vi "casg.vi"(0 "IP adress":string="192.109.209.229", 1 "stop":bool, 2 "Channel":u8(ring)=1 items=["1", "2", "3", "4", "5", "6", "7", "8", "9", "10", "11", "12", "13", "14", "15", "16"], 4 "Exit":bool, 5 "Start":bool, 6 "Draw":enum16{"Ewe(t)", "I(t)"}(ring)) -> (7 "XY Graph":cluster{"Data 101":sgl[], "Data 101":sgl[]}(graph)={"Data 101"=[0.0, 0.01, 0.02, 0.03, 0.04, 0.049999997, 0.06, 0.07, 0.08, 0.089999996, 0.099999994, 0.11, 0.12, 0.13, 0.14, 0.14999999, 0.16, 0.17, 0.17999999, 0.19, 0.19999999, 0.21, 0.22, 0.22999999, 0.24, 0.25, 0.26, 0.26999998, 0.28, 0.29, 0.29999998, 0.31, 0.32, 0.32999998, 0.34, 0.35, 0.35999998, 0.37, 0.38, 0.39, 0.39999998, 0.41, 0.42, 0.42999998, 0.44, 0.45, 0.45999998, 0.47, 0.48, 0.48999998, 0.5, 0.51, 0.52, 0.53, 0.53999996, 0.55, 0.56, 0.57, 0.58, 0.59, 0.59999996, 0.61, 0.62, 0.63, 0.64, 0.65, 0.65999997, 0.66999996, 0.68, 0.69, 0.7, 0.71, 0.71999997, 0.72999996, 0.74, 0.75, 0.76, 0.77, 0.78, 0.78999996, 0.79999995, 0.81, 0.82, 0.83, 0.84, 0.84999996, 0.85999995, 0.87, 0.88, 0.89, 0.9, 0.90999997, 0.91999996, 0.92999995, 0.94, 0.95, 0.96, 0.96999997, 0.97999996, 0.98999995, 1.0, 1.01, 1.02, 1.03, 1.04, 1.05, 1.06, 1.0699999, 1.0799999, 1.0899999, 1.1, 1.11, 1.12, 1.13, 1.14, 1.15, 1.16, 1.17, 1.18, 1.1899999, 1.1999999, 1.2099999, 1.22, 1.23, 1.24, 1.25, 1.26, 1.27, 1.28, 1.29, 1.3, 1.31, 1.3199999, 1.3299999, 1.3399999, 1.35, 1.36, 1.37, 1.38, 1.39, 1.4, 1.41, 1.42, 1.43, 1.4399999, 1.4499999, 1.4599999, 1.4699999, 1.48, 1.49, 1.5, 1.51, 1.52, 1.53, 1.54, 1.55, 1.56, 1.5699999, 1.5799999, 1.5899999, 1.5999999, 1.61, 1.62, 1.63, 1.64, 1.65, 1.66, 1.67, 1.68, 1.6899999, 1.6999999, 1.7099999, 1.7199999, 1.7299999, 1.74, 1.75, 1.76, 1.77, 1.78, 1.79, 1.8, 1.81, 1.8199999, 1.8299999, 1.8399999, 1.8499999, 1.8599999, 1.87, 1.88, 1.89, 1.9, 1.91, 1.92, 1.93, 1.9399999, 1.9499999, 1.9599999, 1.9699999, 1.9799999, 1.9899999, 2.0, 2.01, 2.02, 2.03, 2.04, 2.05, 2.06, 2.07, 2.08, 2.09, 2.1, 2.11, 2.12, 2.1299999, 2.1399999, 2.1499999, 2.1599998, 2.1699998, 2.1799998, 2.19, 2.2, 2.21, 2.22, 2.23, 2.24, 2.25, 2.26, 2.27, 2.28, 2.29, 2.3, 2.31, 2.32, 2.33, 2.34, 2.35, 2.36, 2.37, 2.3799999, 2.3899999, 2.3999999, 2.4099998, 2.4199998, 2.4299998, 2.44, 2.45, 2.46, 2.47, 2.48, 2.49, 2.5, 2.51, 2.52, 2.53, 2.54, 2.55, 2.56, 2.57, 2.58, 2.59, 2.6, 2.61, 2.62, 2.6299999, 2.6399999, 2.6499999, 2.6599998, 2.6699998, 2.6799998, 2.6899998, 2.7, 2.71, 2.72, 2.73, 2.74, 2.75, 2.76, 2.77, 2.78, 2.79, 2.8, 2.81, 2.82, 2.83, 2.84, 2.85, 2.86, 2.87, 2.8799999, 2.8899999, 2.8999999, 2.9099998, 2.9199998, 2.9299998, 2.9399998, 2.9499998, 2.96, 2.97, 2.98, 2.99, 3.0], "Data 101"=array[301 elements]}, 8 "Number of points":i32=301)   [LabVIEW 2014]
uses:
  LLB/dll_Functions.llb/CASGParameters.ctl
panel:
  in  "Display Parameters?":bool caption="Display Parameters"
  out "DllPath":path caption="DLL Path"
  out "LibVersion":string caption="DLL Version"
  in  "CASG Parameters":T1={"Ii"=0.0, "Ii_vs_initial"=TRUE, "Steps"=[{"I1_vs_initial"=FALSE, "I1"=0.0005, "Period_number"=3, "Fs"=1.0, "Record_every_dE"=1.0, "Record_every_dT"=0.01, "I2_vs_initial"=TRUE, "I2"=0.0}, {"I1_vs_initial"=FALSE, "I1"=0.002, "Period_number"=4, "Fs"=10.0, "Record_every_dE"=0.1, "Record_every_dT"=0.001, "I2_vs_initial"=TRUE, "I2"=0.0}], "Step_number"=1, "N_Cycles"=0, "I_Range"=8, "Bandwidth"=5, "em"=1, "ce"=0, "tb"=5e-05} {"tb" min=5e-05 max=1 format="%^_3e"; "Step_number" min=0 max=99; "Steps"."I2" min=-150 max=150 format="%^_3e"; "Steps"."Record_every_dT" min=0 format="%.2e"; "Steps"."Record_every_dE" min=0 format="%.2e"; "Steps"."Fs" min=1e-05 max=1000000 format="%.2e"; "Steps"."Period_number" min=1; "Steps"."I1" min=-150 max=150 format="%^_3e"; "ce" items=["Standard", "CE to ground"]; "Ii" min=-10 max=10 format="%.5f"; "I_Range" items=["1pA", "1nA", "10nA", "100nA", "1µA", "10µA", "100µA", "1mA", "10mA", "100mA", "1A", "Booster"]; "Bandwidth" items=["1"=1, "2"=2, "3"=3, "4"=4, "5"=5, "6"=6, "7"=7, "8"=8, "9"=9]; "N_Cycles" min=0 max=1000 step=1}
  out "Exit 2":bool=TRUE
  out "Data 169":sgl[][](array[numeric])=[[0.0, 0.0009888702, 0.0, 1.0], [0.01, 0.036624238, 3.9297032e-05, 1.0], [0.02, 0.06807284, 6.7561894e-05, 1.0], [0.03, 0.09920054, 0.000100410245, 1.0], [0.04, 0.13097005, 0.00013096684, 1.0], [0.049999997, 0.15985142, 0.00016075955, 1.0], [0.06, 0.1896955, 0.00018902442, 1.0], [0.07, 0.21889777, 0.00021958101, 1.0], [0.08, 0.24681643, 0.00024708195, 1.0], [0.089999996, 0.27345148, 0.00027611072, 1.0], [0.099999994, 0.29976562, 0.00029826426, 1.0], [0.11, 0.32351252, 0.0003250013, 1.0], [0.12, 0.3475803, 0.00034791877, 1.0], [0.13, 0.37100634, 0.00037083623, 1.0], [0.14, 0.3905815, 0.00039069803, 1.0], [0.14999999, 0.41015664, 0.00041132374, 1.0], [0.16, 0.42748544, 0.00042889378, 1.0], [0.17, 0.44353065, 0.00044493595, 1.0], [0.17999999, 0.45893404, 0.0004609782, 1.0], [0.19, 0.4704866, 0.00047396476, 1.0], [0.19999999, 0.48236004, 0.00048313173, 1.0], [0.21, 0.49070355, 0.0004892431, 1.0], [0.22, 0.49712163, 0.0004999379, 1.0], [0.22999999, 0.50193524, 0.00050222967, 1.0], [0.24, 0.50514424, 0.0005068131, 1.0], [0.25, 0.50546515, 0.0005060492, 1.0], [0.26, 0.5045025, 0.00050452136, 1.0], [0.26999998, 0.5012934, 0.0005029935, 1.0], [0.28, 0.49615893, 0.00049917394, 1.0], [0.29, 0.48974085, 0.0004892431, 1.0], [0.29999998, 0.48171824, 0.0004846596, 1.0], [0.31, 0.4708075, 0.00047396476, 1.0], [0.32, 0.45861316, 0.00045868644, 1.0], [0.32999998, 0.44417247, 0.0004456999, 1.0], [0.34, 0.42844817, 0.00043042158, 1.0], [0.35, 0.41047752, 0.00041132374, 1.0], [0.35999998, 0.39026058, 0.00039146192, 1.0], [0.37, 0.37100634, 0.00037083623, 1.0], [0.38, 0.34725943, 0.0003486827, 1.0], [0.39, 0.32479614, 0.00032576523, 1.0], [0.39999998, 0.2988029, 0.00030131993, 1.0], [0.41, 0.27441418, 0.00027687466, 1.0], [0.42, 0.24777915, 0.00024860978, 1.0], [0.42999998, 0.21953958, 0.00021881709, 1.0], [0.44, 0.1900164, 0.00018978832, 1.0], [0.45, 0.16017233, 0.00015999563, 1.0], [0.45999998, 0.13129096, 0.00013173078, 1.0], [0.47, 0.10016325, 0.00010346591, 1.0], [0.48, 0.06871465, 6.8325804e-05, 1.0], [0.48999998, 0.036624238, 3.8533115e-05, 1.0], [0.5, 0.0058174427, 7.212594e-06, 1.0], [0.51, -0.025310256, -2.334401e-05, 1.0], [0.52, -0.056758855, -5.542844e-05, 1.0], [0.53, -0.08788655, -8.674896e-05, 1.0], [0.53999996, -0.11805154, -0.000117305564, 1.0], [0.55, -0.14853743, -0.00014862607, 1.0], [0.56, -0.1780606, -0.00017765485, 1.0], [0.57, -0.20758379, -0.00020668362, 1.0], [0.58, -0.23582333, -0.00023265673, 1.0], [0.59, -0.26245838, -0.00026092157, 1.0], [0.59999996, -0.28748888, -0.0002861308, 1.0], [0.61, -0.31348214, -0.0003128678, 1.0], [0.62, -0.3362663, -0.0003365492, 1.0], [0.63, -0.3596923, -0.0003571749, 1.0], [0.64, -0.37990928, -0.00037627274, 1.0], [0.65, -0.39852172, -0.00039689848, 1.0], [0.65999997, -0.41552964, -0.00041523244, 1.0], [0.66999996, -0.43189573, -0.00043051073, 1.0], [0.68, -0.44665733, -0.0004450251, 1.0], [0.69, -0.45917258, -0.00045724778, 1.0], [0.7, -0.46912062, -0.00046794256, 1.0], [0.71, -0.4774641, -0.00047787346, 1.0], [0.71999997, -0.4851658, -0.0004839848, 1.0], [0.72999996, -0.4899794, -0.0004893322, 1.0], [0.74, -0.49415115, -0.00049162394, 1.0], [0.75, -0.49447203, -0.0004931517, 1.0], [0.76, -0.49447203, -0.00049086, 1.0], [0.77, -0.49062118, -0.0004893322, 1.0], [0.78, -0.48484492, -0.00048322088, 1.0], [0.78999996, -0.47874773, -0.00047940132, 1.0], [0.79999995, -0.47040424, -0.00046870648, 1.0], [0.81, -0.4588517, -0.00045801167, 1.0], [0.82, -0.44665733, -0.00044578905, 1.0], [0.83, -0.43317935, -0.00043203856, 1.0], [0.84, -0.41681325, -0.00041446852, 1.0], [0.84999996, -0.3991635, -0.0003984263, 1.0], [0.85999995, -0.3802302, -0.0003785645, 1.0], [0.87, -0.35937142, -0.0003587027, 1.0], [0.88, -0.33754992, -0.0003334935, 1.0], [0.89, -0.31444484, -0.0003121039, 1.0], [0.9, -0.2884516, -0.0002876586, 1.0], [0.90999997, -0.26310018, -0.0002616855, 1.0], [0.91999996, -0.23550244, -0.00023494849, 1.0], [0.92999995, -0.20758379, -0.0002059197, 1.0], [0.94, -0.17870241, -0.00017841876, 1.0], [0.95, -0.15014194, -0.00014938999, 1.0], [0.96, -0.11901425, -0.000117305564, 1.0], [0.96999997, -0.08884926, -8.598504e-05, 1.0], [0.97999996, -0.05643795, -5.6192355e-05, 1.0], [0.98999995, -0.025952064, -2.487184e-05, 1.0], [1.0, 0.0058174427, 6.448679e-06, 1.0], [1.01, 0.036303334, 3.8533115e-05, 1.0], [1.02, 0.06711013, 6.908972e-05, 1.0], [1.03, 0.09952144, 0.000100410245, 1.0], [1.04, 0.12936553, 0.00012943902, 1.0], [1.05, 0.16049322, 0.00016075955, 1.0], [1.06, 0.1893746, 0.00019055224, 1.0], [1.0699999, 0.21857686, 0.00022034491, 1.0], [1.0799999, 0.24521191, 0.0002478459, 1.0], [1.0899999, 0.27345148, 0.0002745829, 1.0], [1.1, 0.30008653, 0.000300556, 1.0], [1.11, 0.32447523, 0.0003250013, 1.0], [1.12, 0.3475803, 0.0003502105, 1.0], [1.13, 0.3700436, 0.00037160012, 1.0], [1.14, 0.39026058, 0.00039146192, 1.0], [1.15, 0.41047752, 0.00041285154, 1.0], [1.16, 0.42716455, 0.00042965767, 1.0], [1.17, 0.44353065, 0.00044646382, 1.0], [1.18, 0.45829225, 0.00045868644, 1.0], [1.1899999, 0.4704866, 0.00047090912, 1.0], [1.1999999, 0.48043463, 0.00048083998, 1.0], [1.2099999, 0.49038264, 0.0004892431, 1.0], [1.22, 0.49712163, 0.00049917394, 1.0], [1.23, 0.50161433, 0.0005014657, 1.0], [1.24, 0.5048233, 0.0005060492, 1.0], [1.25, 0.506107, 0.0005060492, 1.0], [1.26, 0.5045025, 0.0005060492, 1.0], [1.27, 0.5012934, 0.00050222967, 1.0], [1.28, 0.49744254, 0.0004953544, 1.0], [1.29, 0.48974085, 0.0004892431, 1.0], [1.3, 0.48203915, 0.00048313173, 1.0], [1.31, 0.4711284, 0.00047243692, 1.0], [1.3199999, 0.45765042, 0.00045792255, 1.0], [1.3299999, 0.44353065, 0.0004456999, 1.0], [1.3399999, 0.42812726, 0.00042889378, 1.0], [1.35, 0.41079843, 0.00041055982, 1.0], [1.36, 0.39090237, 0.00039222583, 1.0], [1.37, 0.37068543, 0.00037236404, 1.0], [1.38, 0.34725943, 0.0003502105, 1.0], [1.39, 0.32543793, 0.00032652915, 1.0], [1.4, 0.2991238, 0.00030131993, 1.0], [1.41, 0.2737724, 0.0002745829, 1.0], [1.42, 0.24649553, 0.0002478459, 1.0], [1.43, 0.21953958, 0.00022034491, 1.0], [1.4399999, 0.1890537, 0.00019131615, 1.0], [1.4499999, 0.16113503, 0.0001638152, 1.0], [1.4599999, 0.13097005, 0.00013020294, 1.0], [1.4699999, 0.10016325, 0.000100410245, 1.0], [1.48, 0.06871465, 6.985364e-05, 1.0], [1.49, 0.03758695, 3.77692e-05, 1.0], [1.5, 0.0058174427, 7.212594e-06, 1.0], [1.51, -0.02563116, -2.4107923e-05, 1.0], [1.52, -0.056758855, -5.542844e-05, 1.0], [1.53, -0.08820745, -8.598504e-05, 1.0], [1.54, -0.11805154, -0.00011806948, 1.0], [1.55, -0.14917924, -0.00014557042, 1.0], [1.56, -0.1780606, -0.00017765485, 1.0], [1.5699999, -0.20662107, -0.0002059197, 1.0], [1.5799999, -0.23486063, -0.00023418457, 1.0], [1.5899999, -0.26277927, -0.00025862985, 1.0], [1.5999999, -0.28748888, -0.0002861308, 1.0], [1.61, -0.3128403, -0.00031133997, 1.0], [1.62, -0.33658722, -0.00033502135, 1.0], [1.63, -0.3577669, -0.00035641095, 1.0], [1.64, -0.37926745, -0.0003785645, 1.0], [1.65, -0.3978799, -0.00039766237, 1.0], [1.66, -0.41681325, -0.00041599633, 1.0], [1.67, -0.43253756, -0.00043203856, 1.0], [1.68, -0.44697824, -0.0004450251, 1.0], [1.6899999, -0.45917258, -0.00045877558, 1.0], [1.6999999, -0.4697624, -0.0004694704, 1.0], [1.7099999, -0.47906864, -0.00047787346, 1.0], [1.7199999, -0.48484492, -0.0004839848, 1.0], [1.7299999, -0.4899794, -0.0004885683, 1.0], [1.74, -0.49383023, -0.00049162394, 1.0], [1.75, -0.49350932, -0.00049391564, 1.0], [1.76, -0.49447203, -0.00049238786, 1.0], [1.77, -0.4899794, -0.00048780435, 1.0], [1.78, -0.48484492, -0.00048474869, 1.0], [1.79, -0.47842684, -0.00047940132, 1.0], [1.8, -0.47040424, -0.00046794256, 1.0], [1.81, -0.4588517, -0.00045953953, 1.0], [1.8199999, -0.44826186, -0.0004450251, 1.0], [1.8299999, -0.43285844, -0.00043127465, 1.0], [1.8399999, -0.41649234, -0.00041676027, 1.0], [1.8499999, -0.39948443, -0.00039460673, 1.0], [1.8599999, -0.37958837, -0.00037780058, 1.0], [1.87, -0.3596923, -0.00035641095, 1.0], [1.88, -0.3362663, -0.000338077, 1.0], [1.89, -0.3128403, -0.00031133997, 1.0], [1.9, -0.2884516, -0.00028918646, 1.0], [1.91, -0.26277927, -0.00026015766, 1.0], [1.92, -0.23646514, -0.00023418457, 1.0], [1.93, -0.20790468, -0.0002059197, 1.0], [1.9399999, -0.1783815, -0.00017841876, 1.0], [1.9499999, -0.14917924, -0.00014938999, 1.0], [1.9599999, -0.11837244, -0.000117305564, 1.0], [1.9699999, -0.08820745, -8.7512875e-05, 1.0], [1.9799999, -0.057721566, -5.4664528e-05, 1.0], [1.9899999, -0.025952064, -2.5635754e-05, 1.0], [2.0, 0.0048547303, 7.212594e-06, 1.0], [2.01, 0.037266046, 3.7005288e-05, 1.0], [2.02, 0.06871465, 6.8325804e-05, 1.0], [2.03, 0.098879635, 9.811849e-05, 1.0], [2.04, 0.12968643, 0.00013249468, 1.0], [2.05, 0.16017233, 0.00016075955, 1.0], [2.06, 0.1896955, 0.00019055224, 1.0], [2.07, 0.21825597, 0.00021958101, 1.0], [2.08, 0.24681643, 0.00024631806, 1.0], [2.09, 0.27280968, 0.000273819, 1.0], [2.1, 0.2991238, 0.0002990282, 1.0], [2.11, 0.32447523, 0.0003242374, 1.0], [2.12, 0.34725943, 0.0003502105, 1.0], [2.1299999, 0.3694018, 0.00036854448, 1.0], [2.1399999, 0.38961875, 0.00039146192, 1.0], [2.1499999, 0.41079843, 0.00040979587, 1.0], [2.1599998, 0.42780635, 0.00043042158, 1.0], [2.1699998, 0.44417247, 0.0004456999, 1.0], [2.1799998, 0.45797133, 0.00045945038, 1.0], [2.19, 0.4698448, 0.00047243692, 1.0], [2.2, 0.48139733, 0.00048389565, 1.0], [2.21, 0.48974085, 0.000490007, 1.0], [2.22, 0.49647984, 0.00049688225, 1.0], [2.23, 0.5022561, 0.00050375744, 1.0], [2.24, 0.5045025, 0.0005060492, 1.0], [2.25, 0.50514424, 0.00050757703, 1.0], [2.26, 0.5048233, 0.0005060492, 1.0], [2.27, 0.5012934, 0.00050375744, 1.0], [2.28, 0.49712163, 0.00049764616, 1.0], [2.29, 0.49038264, 0.0004915348, 1.0], [2.3, 0.48011371, 0.00048389565, 1.0], [2.31, 0.4708075, 0.00047243692, 1.0], [2.32, 0.45797133, 0.00045945038, 1.0], [2.33, 0.44385156, 0.00044493595, 1.0], [2.34, 0.42716455, 0.00042812986, 1.0], [2.35, 0.41047752, 0.00041055982, 1.0], [2.36, 0.39122328, 0.00039298975, 1.0], [2.37, 0.37100634, 0.00037236404, 1.0], [2.3799999, 0.34790123, 0.00034791877, 1.0], [2.3899999, 0.32415432, 0.00032652915, 1.0], [2.3999999, 0.30008653, 0.000300556, 1.0], [2.4099998, 0.2740933, 0.000273819, 1.0], [2.4199998, 0.24681643, 0.0002478459, 1.0], [2.4299998, 0.21825597, 0.00021958101, 1.0], [2.44, 0.1900164, 0.00019055224, 1.0], [2.45, 0.15985142, 0.00016305129, 1.0], [2.46, 0.13032824, 0.00013020294, 1.0], [2.47, 0.09984235, 0.00010117416, 1.0], [2.48, 0.06871465, 6.679798e-05, 1.0], [2.49, 0.038228758, 3.8533115e-05, 1.0], [2.5, 0.0051756343, 6.448679e-06, 1.0], [2.51, -0.02498935, -2.334401e-05, 1.0], [2.52, -0.05643795, -5.6192355e-05, 1.0], [2.53, -0.08852836, -8.8276785e-05, 1.0], [2.54, -0.118693344, -0.00011654164, 1.0], [2.55, -0.14821652, -0.00014633434, 1.0], [2.56, -0.1780606, -0.00017459918, 1.0], [2.57, -0.20694198, -0.00020668362, 1.0], [2.58, -0.23550244, -0.00023418457, 1.0], [2.59, -0.26149565, -0.00026092157, 1.0], [2.6, -0.2878098, -0.00028995035, 1.0], [2.61, -0.3125194, -0.0003121039, 1.0], [2.62, -0.3359454, -0.00033578524, 1.0], [2.6299999, -0.3590505, -0.00035641095, 1.0], [2.6399999, -0.37894657, -0.00037627274, 1.0], [2.6499999, -0.3988426, -0.00039689848, 1.0], [2.6599998, -0.41552964, -0.00041523244, 1.0], [2.6699998, -0.43189573, -0.00043051073, 1.0], [2.6799998, -0.44762003, -0.00044731685, 1.0], [2.6899998, -0.4598144, -0.00045877558, 1.0], [2.7, -0.46912062, -0.00046794256, 1.0], [2.71, -0.47842684, -0.00047710957, 1.0], [2.72, -0.4851658, -0.00048322088, 1.0], [2.73, -0.491263, -0.0004885683, 1.0], [2.74, -0.49350932, -0.0004931517, 1.0], [2.75, -0.49511385, -0.00049391564, 1.0], [2.76, -0.49286753, -0.00049238786, 1.0], [2.77, -0.4919048, -0.0004900961, 1.0], [2.78, -0.4851658, -0.0004839848, 1.0], [2.79, -0.47842684, -0.00047863738, 1.0], [2.8, -0.47040424, -0.0004694704, 1.0], [2.81, -0.45853078, -0.00045953953, 1.0], [2.82, -0.44729912, -0.00044578905, 1.0], [2.83, -0.43253756, -0.00043356637, 1.0], [2.84, -0.41777596, -0.00041446852, 1.0], [2.85, -0.3988426, -0.00039689848, 1.0], [2.86, -0.3802302, -0.0003785645, 1.0], [2.87, -0.3596923, -0.00035793878, 1.0], [2.8799999, -0.33787084, -0.0003334935, 1.0], [2.8899999, -0.31444484, -0.0003121039, 1.0], [2.8999999, -0.2884516, -0.00028842254, 1.0], [2.9099998, -0.26181656, -0.00026092157, 1.0], [2.9199998, -0.23518153, -0.00023418457, 1.0], [2.9299998, -0.20726287, -0.0002059197, 1.0], [2.9399998, -0.17934422, -0.00017841876, 1.0], [2.9499998, -0.14950013, -0.00014862607, 1.0], [2.96, -0.119656056, -0.00011501381, 1.0], [2.97, -0.08884926, -8.522113e-05, 1.0], [2.98, -0.05707976, -5.3136693e-05, 1.0], [2.99, -0.025952064, -2.487184e-05, 1.0], [3.0, 0.004533826, 5.684764e-06, 1.0]] format="%.2f"
  # "Instructions:\nBefore running the VI you must type a valid IP adress that corresponds to the instrument.Then press the Run button to execute this VI.\nWhile this VI is running, choose the available channel, enter the CASG parameters or keep the default values, then press the start button to begin the experience.\nChoose the waveform to draw (Ewe(t) or I(t)). You can stop the measure if you press the stop button and exit the execution if you press the exit button."
  # "Set Ii (A)  vs. previous"
  # "repeat nc times"
  # "with I Range"
  # "bandwidth"
  # "Fs (Hz)"
  # "record every dE (V)"
  # "or every dt (s)"
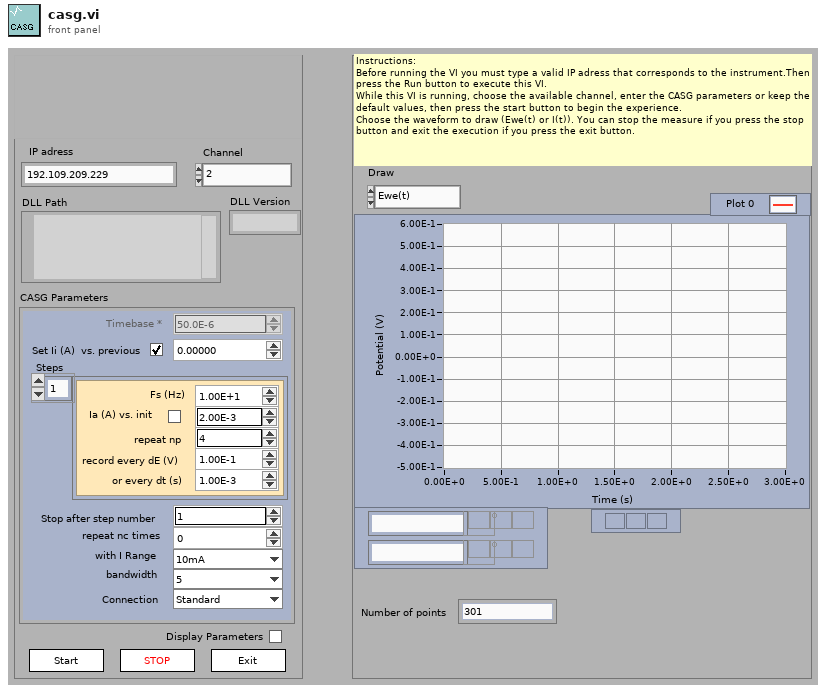
[diagram p1: front panel]
types:
  T1 = typedef "CASGParameters.ctl" = cluster{"Ii":sgl, "Ii_vs_initial":bool, "Steps":cluster{"I1_vs_initial":bool, "I1":sgl, "Period_number":u32, "Fs":sgl, "Record_every_dE":sgl, "Record_every_dT":sgl, "I2_vs_initial":bool, "I2":sgl}[], "Step_number":i32, "N_Cycles":i32, "I_Range":u16, "Bandwidth":u16, "em":u16, "ce":u16, "tb":sgl}
  T2 = cluster{"LibVersion":string, "StringLength":u32, "DllPath":path}
  T3 = cluster{"Channel":i32, "BoardVersion":i32, "BoardSerialCode":i32, "FirmwareCode":i32, "FirmwareVersion":i32, "XilinxVersion":i32, "AmpCode":i32, "NbAmp":i32, "LcBoard":i32, "Zboard":i32, "MuxBoard":i32, "GPRAboard":i32, "MemSize":i32, "MemFilled":i32, "state":i32, "MaxIRange":i32, "MinIRange":i32, "MaxBandwidth":i32, "NbOfTechniques":i32}
  T4 = typedef "TechniqueParameters.ctl" = cluster{"String Label":string, "Type":i32, "Valeur":i32, "Index":i32}
  T5 = cluster{"string before end tag":string, i32, i32, i32}[]
  T6 = cluster{"IRQskipped":i32, "NbRaws":i32, "NbCols":i32, "Technique Index":i32, "TechniqueID":i32, "PrcessIndex":i32, "loop":i32, "StartTime":dbl, "MuxPad":i32}
  T7 = cluster{"State":i32, "MemFilled":i32, "TimeBase":sgl, " Ewe":sgl, " EweRangeMin":sgl, " EweRangeMax":sgl, "Ece":sgl, "EceRangeMin":sgl, "EceRangeMax":sgl, "Eoverflow":i32, "I":sgl, "IRange":i32, "Ioverflow":i32, "ElapsedTime":sgl, "Freq":sgl, "Rcomp":sgl, "Saturation":sgl, "OptErr":i32, "OptPos":i32}
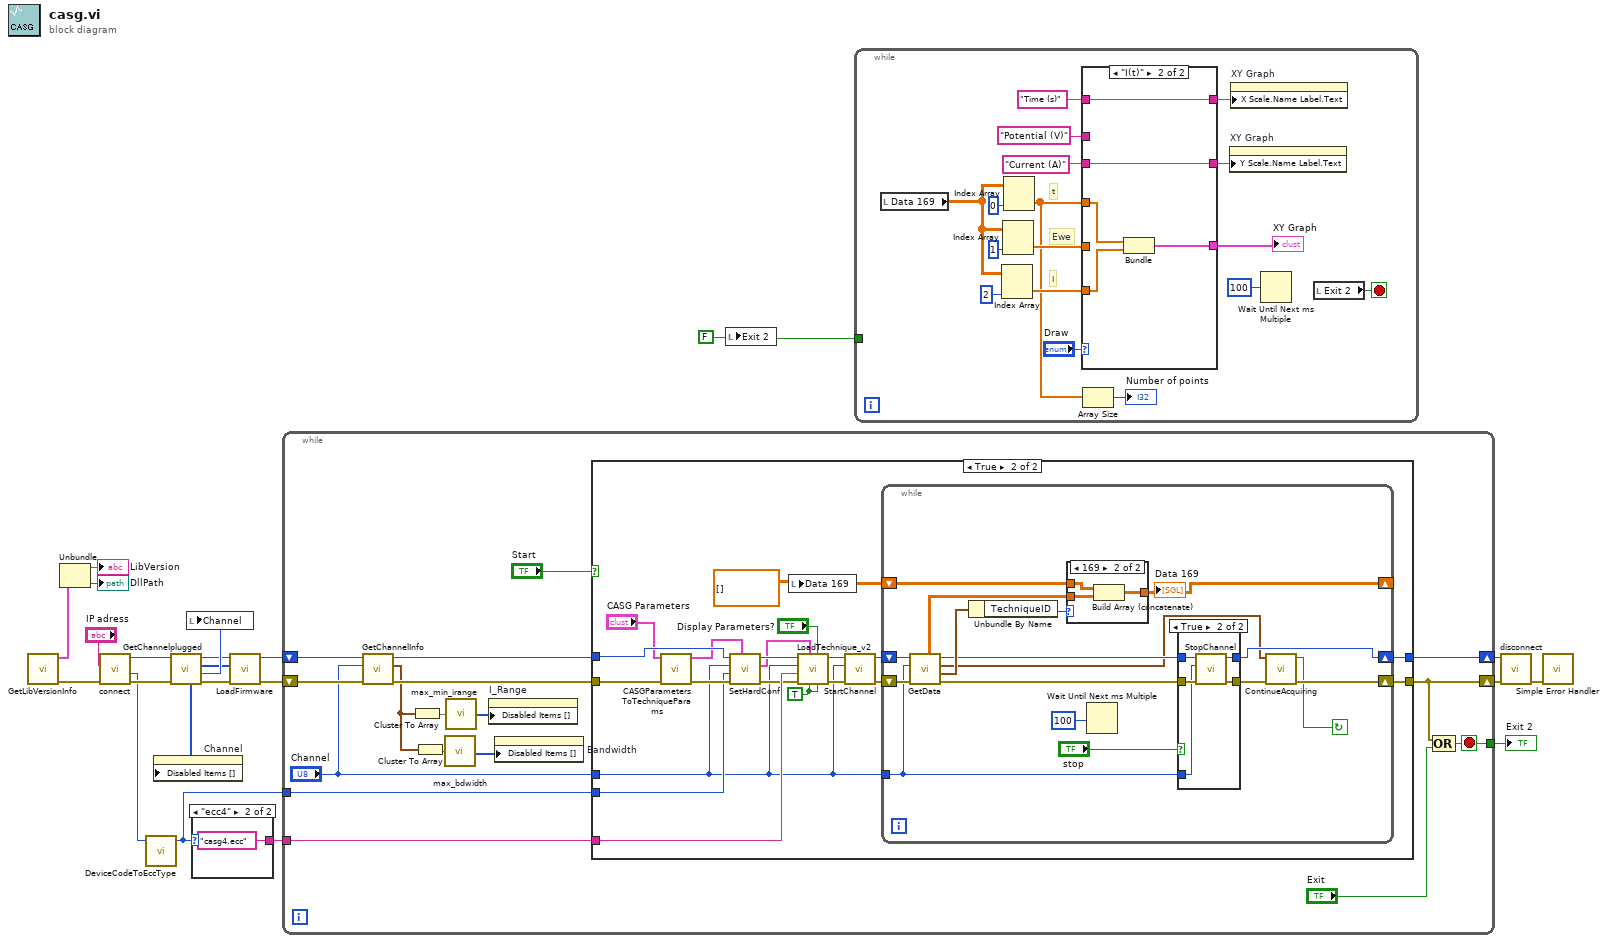
[diagram p0: block diagram]
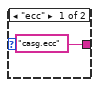
[diagram p2: hidden frame]
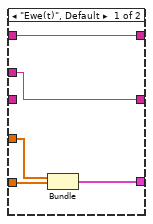
[diagram p3: hidden frame]
diagram:
  w21 = FALSE ("Exit 2")
  n1 = call "GetLibVersionInfo.vi"() -> ("error out"=w1:errorcluster, "LibInfo"=w4:T2)  [unwired: 10 in]
  n2 = Unbundle(w4) -> ("LibVersion"=→"LibVersion":string, "DllPath"=→"DllPath":path)  [unwired: 1 out]
  n3 = call "connect.vi"("error in (no error)"=w1, "IP"="IP adress") -> ("error out"=w17:errorcluster, "Device Code"=w7:i32, "ID Out"=w13:i32)  [unwired: 6 in, 1 out]
  n4 = call "DeviceCodeToEccType.vi"("Device Code"=w7) -> ("EccType"=w5:enum16{"ecc", "ecc4"})  [unwired: 4 in]
  n5 = call "GetChannelplugged.vi"("error in (no error)"=w17, "ID In"=w13) -> ("error out"=w16:errorcluster, "FirstPluggedChannel"=w19:u8, "PluggedChannels"=w10:u8[], "ID Out"=w12:i32, "DisabledChannels"=w14:i32[])  [unwired: 5 in]
  n6 = property on="Channel" class="Ring (strict)"("Disabled Items []"=w14) -> ()  [unwired: 2 in, 2 out]
  n7 = local write "Channel"(w19) -> ()
  n8 = case shown="\"ecc4\"" w5 {
    tunnel: ["casg.ecc" ("FName") "casg4.ecc" ("FName")] -> w6
    frame "ecc" {
    }
    frame "ecc4" {
    }
  }
  n9 = call "LoadFirmware.vi"("error in (no error)"=w16, "Channels"=w10, "ID In"=w12) -> ("error out"=w15:errorcluster, "ID Out"=w11:i32)  [unwired: 6 in, 1 out]
  n10 = while {
    shift-right: [w28] -> w9
    shift-left: w15 -> [w35]
    tunnel: [w26] -> w22
    shift-right: [w38] -> w18
    shift-left: w11 -> [w31]
    tunnel: w6 -> [w29]
    tunnel: w5 -> [w25]
    stop <- w26 stop-if-true
    n11 = call "GetChannelInfo.vi"("error in (no error)"=w35, "Channel"="Channel", "ID"=w31) -> ("error out"=w34:errorcluster, "Channel information"=w33:T3, "ID Out"=w30:i32)  [unwired: 6 in]
    n12 = Cluster To Array(cluster=w33) -> (array=w40:i32[])
    n13 = Cluster To Array(cluster=w33) -> (array=w39:i32[])
    n14 = call "max_bdwidth.vi"("resources"=w39) -> ("disabled ranges"=w36:i32[])
    n15 = call "max_min_irange.vi"("resources"=w40) -> ("disabled ranges"=w37:i32[])
    n16 = property on="I_Range" class="Ring (strict)"("Disabled Items []"=w37) -> ()  [unwired: 2 in, 2 out]
    n17 = property on="Bandwidth" class="Ring (strict)"("Disabled Items []"=w36) -> ()  [unwired: 2 in, 2 out]
    n18 = case shown="True" "Start" {
      tunnel: "Channel" -> [_ w46]
      tunnel: [w43 w63] -> w28
      tunnel: w34 -> [w43 w60]
      tunnel: w30 -> [w42 w52]
      tunnel: [w42 w55] -> w38
      tunnel: w29 -> [_ w54]
      tunnel: w25 -> [_ w47]
      frame False {
      }
      frame True {
        w59 = TRUE ("First Protocol")
        w62 = sgl[][] []
        n19 = call "CASGParametersToTechniqueParams.vi"("error in (no error)"=w60, "CASG  Parameters"="CASG Parameters") -> ("error out"=w53:errorcluster, "TechniquesParameters"=w50:T4[])  [unwired: 8 in]
        n20 = call "SetHardConf.vi"("Params Values"=w50, "error in (no error)"=w53, "EccType"=w47, "Channel"=w46, "ID In"=w52) -> ("error out"=w48:errorcluster, "Params Values Trimed"=w45:T5, "ID Out"=w49:i32)  [unwired: 4 in]
        n21 = local write "Data 169"(w62) -> ()
        n22 = call "LoadTechnique_v2.vi"("Last Protocol"=w59, "Display Parameters?"="Display Parameters?", "First Protocol"=w59, "TechniqueParameters"=w45, "error in (no error)"=w48, "FName"=w54, "Selected Channel"=w46, "ID In"=w49) -> ("error out"=w58:errorcluster, "ID  Out"=w57:i32)  [unwired: 2 in]
        n23 = call "StartChannel.vi"("error in (no error)"=w58, "Channel"=w46, "ID In"=w57) -> ("error out"=w61:errorcluster, "ID Out"=w56:i32)  [unwired: 7 in]
        n24 = while {
          shift-right: [w67] -> w63
          shift-left: w61 -> [w80]
          shift-right: [w77] -> _
          shift-left: w62 -> [w78]
          tunnel: w46 -> [w74]
          shift-right: [w68] -> w55
          shift-left: w56 -> [w70]
          stop <- w65 continue-if-true
          n25 = call "GetData.vi"("error in (no error)"=w80, "Channel"=w74, "ID In"=w70) -> ("error out"=w76:errorcluster, "Data information"=w73:T6, "Current values"=w64:T7, "ID Out"=w69:i32, "Data"=w71:dbl[][])  [unwired: 4 in]
          n26 = Unbundle By Name(w73) -> ("TechniqueID"=w72:i32)
          n27 = case shown="169" w72 {
            tunnel: w71 -> [_ w91]
            tunnel: w78 -> [w88 w90]
            tunnel: [w88 w89] -> w77
            frame 0, Default {
            }
            frame 169 {
              n28 = Build Array (concatenate)(w90, w91) -> (w89:dbl[][])
            }
          }
          "Data 169" <- w77
          n29 = Wait Until Next ms Multiple(millisecond multiple=u32 100) -> ()  [unwired: 1 out]
          n30 = case shown="True" "stop" {
            tunnel: [w82 w87] -> w66
            tunnel: w76 -> [w82 w86]
            tunnel: w74 -> [_ w85]
            tunnel: w69 -> [w81 w84]
            tunnel: [w81 w83] -> w68
            frame False {
            }
            frame True {
              n31 = call "StopChannel.vi"("error in (no error)"=w86, "Channel"=w85, "ID In"=w84) -> ("error out"=w87:errorcluster, "ID Out"=w83:i32)  [unwired: 7 in]
            }
          }
          n32 = call "ContinueAcquiring.vi"("error in"=w66, "Current values"=w64) -> ("error out"=w67:errorcluster, "ContinueAcquiring?"=w65:bool)  [unwired: 8 in]
        }
      }
    }
    n33 = Compound Arithmetic op=OR(w28, "Exit") -> (w26:bool)
  }
  "Exit 2" <- w22
  n34 = local write "Exit 2"(w21) -> ()
  n35 = while {
    tunnel: w21 -> [_]
    stop <- w107 stop-if-true
    # "I"
    # "Ewe"
    # "t"
    n36 = local read "Data 169"() -> (w96:sgl[][])
    n37 = Index Array(array=w96, index (col)=2 ("indice désactivé (col)")) -> (element=w93:sgl[])  [unwired: 1 in]
    n38 = Index Array(array=w96, index (col)=1 ("Index")) -> (element=w95:sgl[])  [unwired: 1 in]
    n39 = Index Array(array=w96, index (col)=0 ("Index")) -> (element=w92:sgl[])  [unwired: 1 in]
    n40 = case shown="\"I(t)\"" "Draw" {
      tunnel: w92 -> [w113 w118]
      tunnel: [w110 w114] -> w94
      tunnel: "Potential (V)" ("Y Scale.Name Label.Text") -> [w112 _]
      tunnel: "Current (A)" ("Y Scale.Name Label.Text") -> [_ w117]
      tunnel: [w112 w117] -> w101
      tunnel: [w111 w116] -> w100
      tunnel: "Time (s)" ("Y Scale.Name Label.Text") -> [w111 w116]
      tunnel: w95 -> [w109 _]
      tunnel: w93 -> [_ w115]
      frame "Ewe(t)", Default {
        n41 = Bundle("Data 169"=w113, "Data 169"=w109) -> (w110:cluster{"Data 169":sgl[], "Data 169":sgl[]})  [unwired: 1 in]
      }
      frame "I(t)" {
        n42 = Bundle("Data 169"=w118, "Data 169"=w115) -> (w114:cluster{"Data 169":sgl[], "Data 169":sgl[]})  [unwired: 1 in]
      }
    }
    "XY Graph" <- w94
    n43 = Array Size(array=w92) -> (size(s)=→"Number of points":i32)
    n44 = property on="XY Graph" class="XYGraph (strict)"("Y Scale.Name Label.Text"=w101) -> ()  [unwired: 2 in, 2 out]
    n45 = property on="XY Graph" class="XYGraph (strict)"("X Scale.Name Label.Text"=w100) -> ()  [unwired: 2 in, 2 out]
    n46 = Wait Until Next ms Multiple(millisecond multiple=u32 100) -> ()  [unwired: 1 out]
    n47 = local read "Exit 2"() -> (w107:bool)
  }
  n48 = call "disconnect.vi"("error in (no error)"=w9, "ID In"=w18) -> ("error out"=w8:errorcluster)  [unwired: 9 in]
  n49 = call <vilib>:"Simple Error Handler.vi"("error in (no error)"=w8) -> ()  [unwired: 4 in, 5 out]
